vi "PNA_SA_SET-FREQ.vi"(0 "Session In":refnum<visa-resource-name>="TCPIP0::K-Instr0000.local::hislip0::INSTR", 5 "error in":errorcluster {"code" format="%.0x"}, 7 "FREQ":dbl=20.0 format="%#_6f", 8 "Timeout":u32=5000, 9 "Units":i64(ring)=1000000000 items=["GHz"=1000000000, "MHZ"=1000000], 10 "RO(T)":bool, 11 "CH":i32=3, 13 "Source":i32=1) -> (12 "freq":dbl=5.0, 14 "Session Out":refnum<visa-resource-name>="TCPIP0::K-Instr0000.local::hislip0::INSTR", 19 "error out":errorcluster {"code" format="%.0x"})   [LabVIEW 2018]
doc: "Applicable Models: All with Spectrum Analysis Options (S9x09xxA/B, S9x09xA/B)\n\n(Read-Write) Set and read the source CW frequency.\n \nParameters\n \n \n<ch>\n Any existing SA channel. If unspecified, value is set to 1.\n \n<port>\n Source port number of the VNA. If unspecified, value is set to 1. To make settings for ports that are not simple numbers, use the [src] argument.\n \n<num>\n CW frequency in Hz. Choose a value within the frequency range of the analyzer.\n \n[,src]\n String. (NOT case sensitive). Source port. Optional. Use SOUR:CAT? to return a list of valid port names.\n\nWhile this argument can be used to make settings for ALL ports, it is designed to access ports such as an external source, or one of the Source 2 outputs on the 2-port 2-source PNA-X model such as \"Port 1 Src2\". Otherwise, the <port> argument performs the same function. If both arguments are specified, [src] takes priority.\n \nExamples\n SENS:SA:SOUR:FREQ:CW 1e10\n\nsense2:sa:source:frequency:cw 1e9,\"Port 1 Src2\"\n \nQuery Syntax\n SENSe<ch>:SA:SOURce<port>:FREQuency:CW?\n \nReturn Type\n Numeric\n \nDefault\n Center frequency of the analyzer"
panel:
  out "concatenated string":string="sens3:sa:sour1:freq:cw?\nsens3:sa:sour1:freq:cw 5000000000.000000\n"
  # "Instrument Address"
  # "Select Source"
  # "Conditions"
  # "Is Read Only (T)"
  # "Channel"
  # "Source"
  # "Inst Timeout(ms)"
  # "Set Freq"
  # "Freq"
  # "Read"
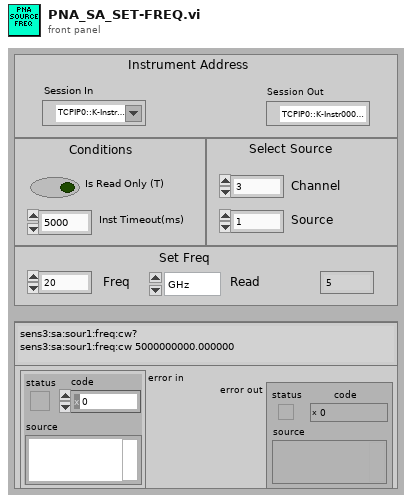
[diagram p1: front panel]
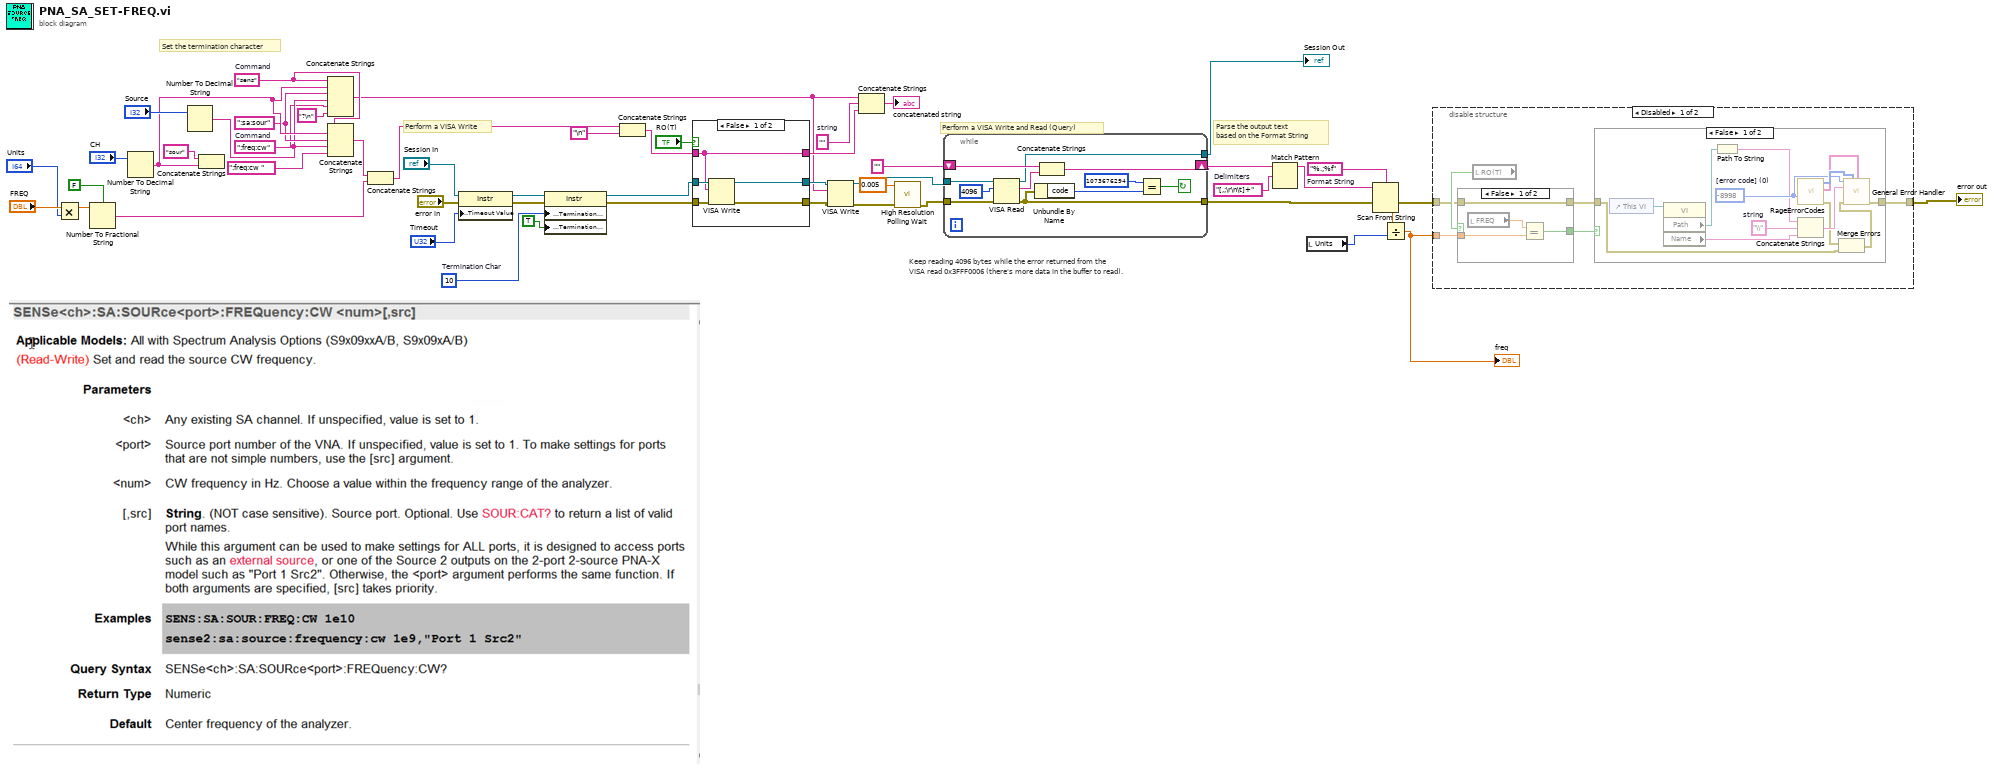
[diagram p0: block diagram]
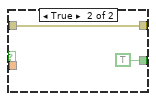
[diagram p2: hidden frame]
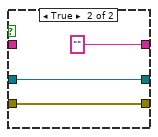
[diagram p5: hidden frame]
diagram:
  w17 = ":sa:sour"  # Command
  w24 = ""  # string
  w30 = "[,;\r\n\t]+"  # Delimiters
  w31 = "%.;%f"  # Format String
  w19 = "sens"  # Command
  w43 = u8 10  # Termination Char
  # "Parse the output text based on the Format String"
  # "Perform a VISA Write and Read (Query)"
  # "Keep reading 4096 bytes while the error returned from the\nVISA read 0x3FFF0006 (there's more data in the buffer to read)."
  # "Perform a VISA Write"
  # "Set the termination character"
  n1 = Multiply(x="FREQ", y="Units") -> (x*y=w13:dbl)
  n2 = Number To Fractional String(use system decimal point (T)=FALSE, number=w13) -> (F-format string=w11:string)  [unwired: 2 in]
  n3 = Number To Decimal String(number="CH") -> (decimal integer string=w18:string)  [unwired: 1 out]
  n4 = Number To Decimal String(number="Source") -> (decimal integer string=w16:string)  [unwired: 1 out]
  n5 = Concatenate Strings("sour" ("staticText"), w18) -> ()  [unwired: 1 out]
  n6 = Concatenate Strings(w19, w18, w17, w16, ":freq:cw" ("Command"), "?\n" ("Command")) -> (w6:string)
  n7 = Concatenate Strings(w19, w18, w17, w16, ":freq:cw " ("Command")) -> (w14:string)
  n8 = Concatenate Strings(w14, w11) -> (w37:string)
  n9 = property class="Instr"(reference="Session In", error in="error in", "General Settings:Timeout Value"="Timeout") -> (reference out=w42:refnum<visa-resource-name>, error out=w45:errorcluster)
  n10 = property class="Instr"(reference=w42, error in=w45, "Message Based Settings:Termination Character"=w43, "Message Based Settings:Termination Character Enable"=TRUE ("enable")) -> (reference out=w29:refnum<visa-resource-name>, error out=w44:errorcluster)
  n11 = Concatenate Strings(w37, "\n" ("StaticText")) -> (w38:string)
  n12 = case shown="False" "RO(T)" {
    tunnel: w44 -> [w56 w58]
    tunnel: [w52 w58] -> w39
    tunnel: w38 -> [w54 _]
    tunnel: w29 -> [w55 w59]
    tunnel: [w53 w59] -> w28
    tunnel: [w54 ""] -> w7
    frame False {
      n13 = VISA Write(VISA resource name=w55, write buffer=w54, error in (no error)=w56) -> (VISA resource name out=w53:refnum<visa-resource-name>, error out=w52:errorcluster)  [unwired: 1 out]
    }
    frame True {
    }
  }
  n14 = VISA Write(VISA resource name=w28, write buffer=w6, error in (no error)=w39) -> (VISA resource name out=w3:refnum<visa-resource-name>, error out=w4:errorcluster)  [unwired: 1 out]
  n15 = Concatenate Strings(w6, w24, w7) -> (→"concatenated string":string)
  n16 = call <vilib>:"High Resolution Polling Wait.vi"("error in (no error)"=w4, "seconds to wait"=0.005) -> ("error out"=w5:errorcluster)  [unwired: 9 in]
  n17 = while {
    tunnel: w3 -> [w67]
    shift-right: [w61] -> w33
    shift-left: "" -> [w66]
    tunnel: w5 -> [w64]
    tunnel: [w63] -> w35
    tunnel: [w60] -> w27
    stop <- w62 continue-if-true
    n18 = VISA Read(VISA resource name=w67, byte count=u32 4096 ("byte count (0)"), error in (no error)=w64) -> (VISA resource name out=w60:refnum<visa-resource-name>, read buffer=w65:string, error out=w63:errorcluster)  [unwired: 1 out]
    n19 = Unbundle By Name(w63) -> ("code"=w69:i32)
    n20 = Concatenate Strings(w66, w65) -> (w61:string)
    n21 = Equal?(x=1073676294, y=w69) -> (x = y?=w62:bool)
  }
  "Session Out" <- w27
  n22 = Match Pattern(string=w33, regular expression=w30) -> (before substring=w32:string)  [unwired: 1 in, 3 out]
  n23 = local read "Units"() -> (w8:i64)
  n24 = Scan From String(format string=w31, input string=w32, error in=w35) -> (error out=w1:errorcluster, output 1=w21:dbl)  [unwired: 2 in, 2 out]
  n25 = Divide(x=w21, y=w8) -> (x/y=w10:dbl)
  "freq" <- w10
  n26 = disable-structure shown="Disabled" {
    disable-tunnel: [w75 w97] -> w22
    disable-tunnel: w10 -> [w74 _]
    disable-tunnel: w1 -> [w72 w97]
    frame Disabled {
      n27 = local read "RO(T)"() -> (w73:bool)
      n28 = case shown="False" w73 {
        tunnel: [w80 TRUE] -> w76
        tunnel: w74 -> [w79 _]
        tunnel: w72 -> [w77 w81]
        tunnel: [w77 w81] -> w71
        frame False {
          n29 = local read "FREQ"() -> (w78:dbl)
          n30 = Equal?(x=w78, y=w79) -> (x = y?=w80:bool)
        }
        frame True {
        }
      }
      n31 = case shown="False" w76 {
        tunnel: w71 -> [w83 w96]
        tunnel: [w95 w96] -> w75
        frame False {
          w86 = "\\"  # string
          w92 = -8998  # [error code] (0)
          n32 = control-ref of="This VI"() -> (w91:refnum<vi>)
          n33 = property class="VI"(reference=w91) -> ("Path"=w89:path, "Name"=w87:string)  [unwired: 1 in, 2 out]
          n34 = Path To String(path=w89) -> (string=w88:string)
          n35 = call "RageErrorCodes.vi"("code"=w92) -> ("error out"=w84:errorcluster, "desc ary"=w93:string[], "code ary"=w94:i32[])  [unwired: 7 in, 1 out]
          n36 = Concatenate Strings(w88, w86, w87) -> (w90:string)
          n37 = Merge Errors(w84, w83) -> (w85:errorcluster)
          n38 = call <vilib>:"General Error Handler.vi"("[error code] (0)"=w92, "[user-defined codes]"=w94, "[user-defined descriptions]"=w93, "[error source] (\" \")"=w90, "error in (no error)"=w85) -> ("error out"=w95:errorcluster)  [unwired: 6 in, 4 out]
        }
        frame True {
        }
      }
    }
    frame Enabled {
    }
  }
  "error out" <- w22
